vi "WPI_CameraIPCameraRead - Copy.vi"(0 "Refnum in":T1, 1 "Operation":enum16{"Read", "Reopen", "Close"}(ring), 2 "port":u16=80, 5 "address":string, 7 "cgi string":string, 11 "error in (no error)":errorcluster, 13 "Authenticate":bool=TRUE) -> (4 "Refnum out":T1, 6 "length":i32, 10 "Reconnect":bool, 15 "error out":errorcluster)   [LabVIEW 2018]
uses:
  <vilib>/vision/Image Controls.llb/IMAQ Image.ctl
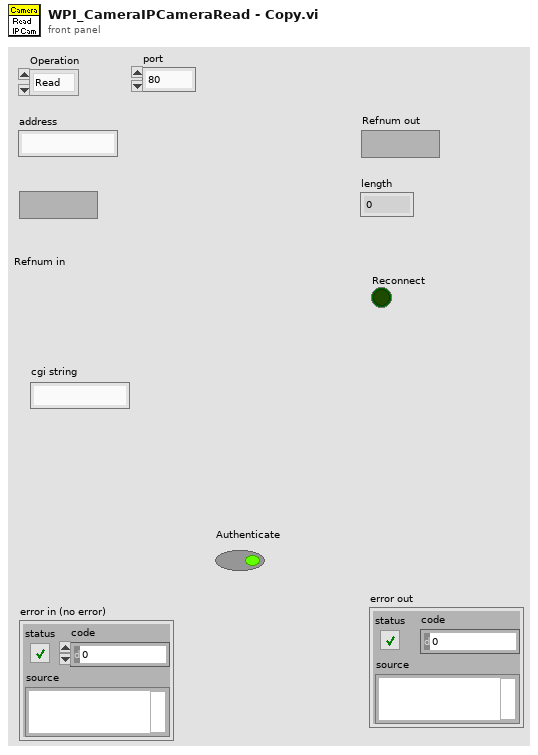
[diagram p1: front panel]
types:
  T1 = typedef "IMAQ Image.ctl" = refnum<image>
  T2 = enum16{"Standard", "Buffered", "CRLF", "Immediate"}
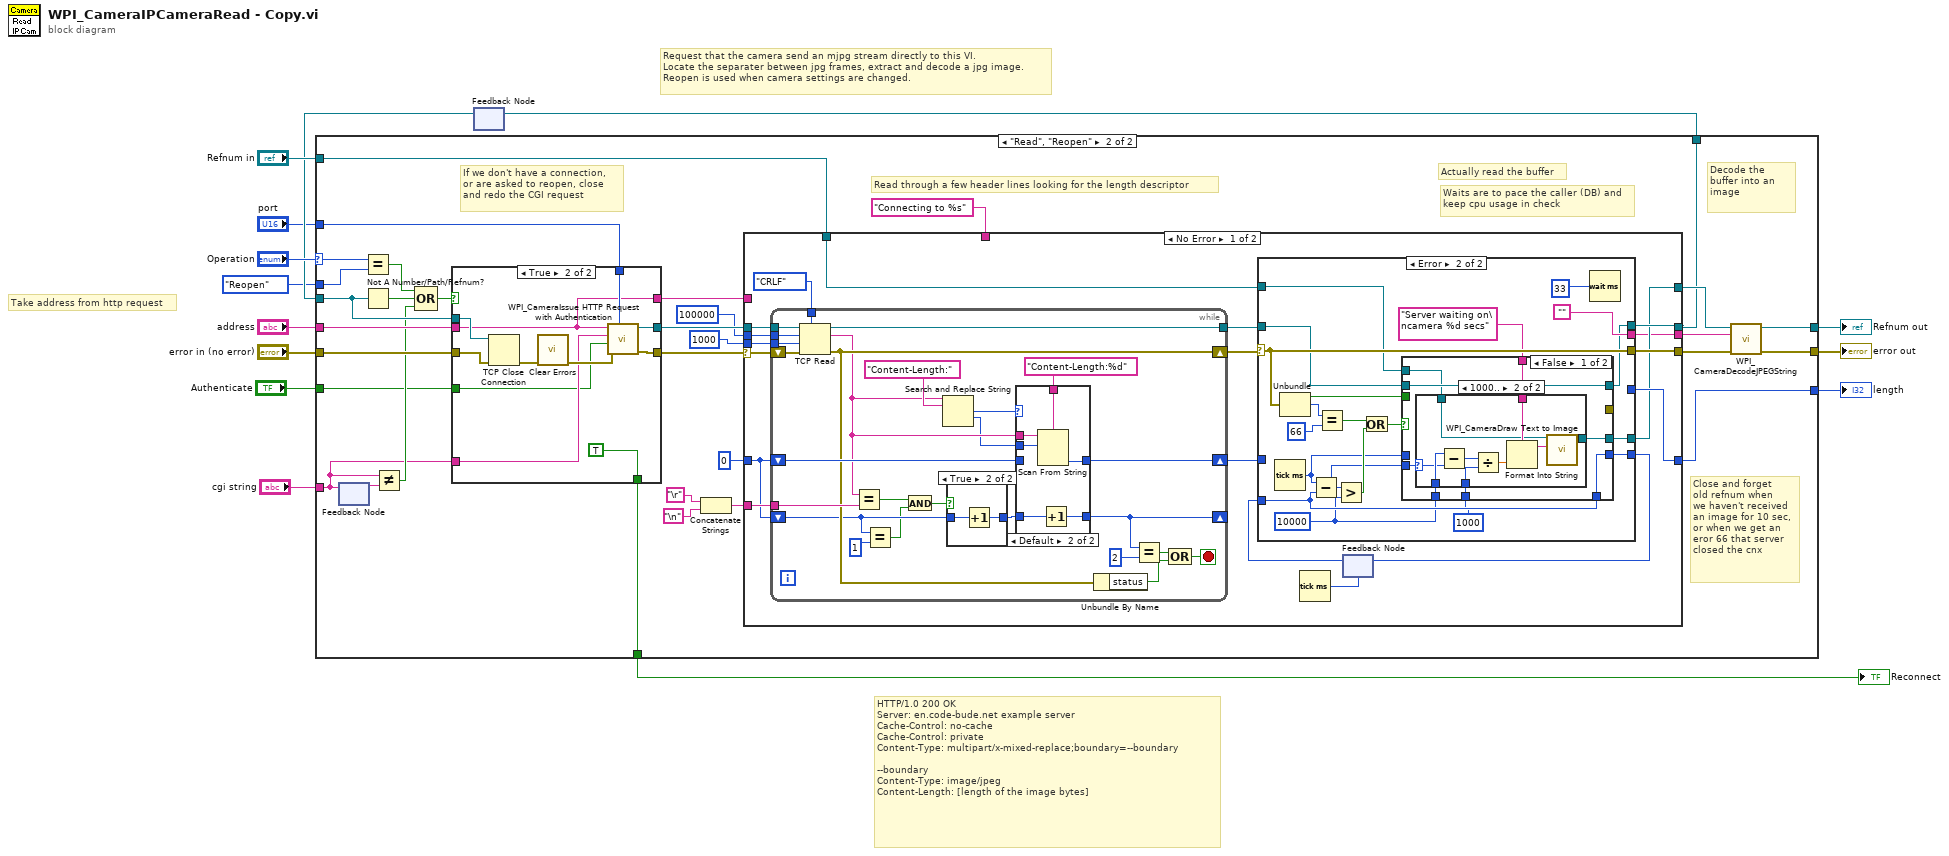
[diagram p0: block diagram]
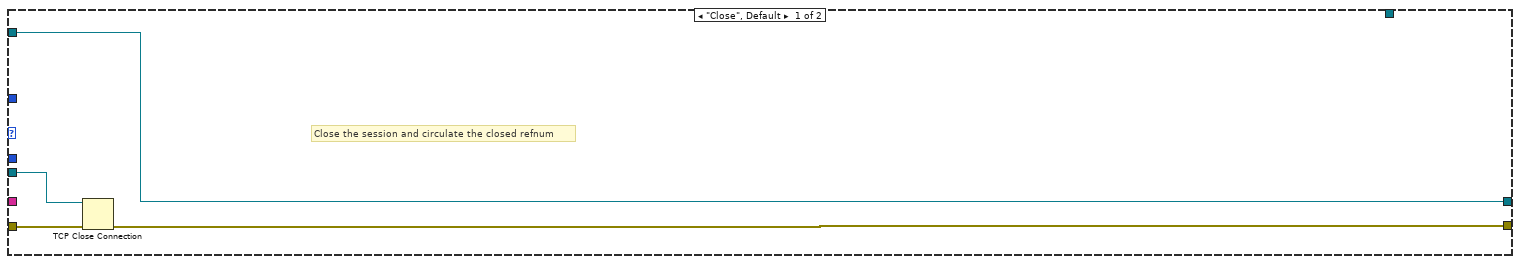
[diagram p2: hidden frame]
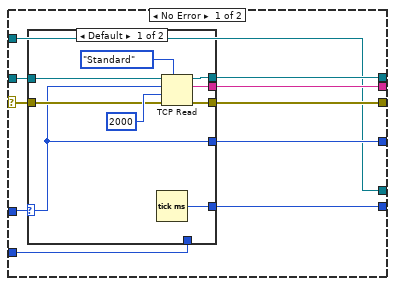
[diagram p4: hidden frame]
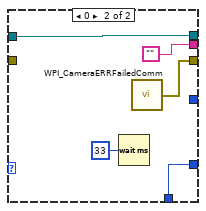
[diagram p5: hidden frame]
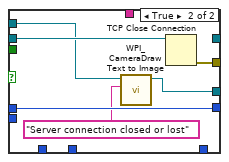
[diagram p7: hidden frame]
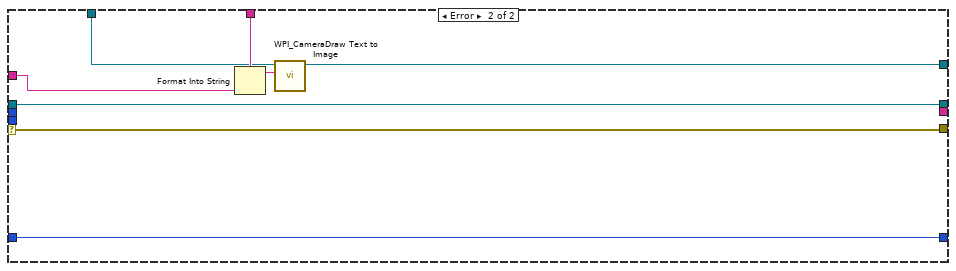
[diagram p10: hidden frame]
diagram:
  # "HTTP/1.0 200 OK\nServer: en.code-bude.net example server\nCache-Control: no-cache\nCache-Control: private\nContent-Type: multipart/x-mixed-replace;boundary=--boundary\n \n--boundary\nContent-Type: image/jpeg\nContent-Length: [length of the image bytes]"
  # "Take address from http request"
  # "Request that the camera send an mjpg stream directly to this VI.\nLocate the separater between jpg frames, extract and decode a jpg image.\nReopen is used when camera settings are changed."
  n1 = feedback #1() -> (w11:refnum<k5>)  [unwired: 1 out]
  n2 = case shown="\"Read\", \"Reopen\"" "Operation" {
    selector: "Operation" -> [_ w38]
    tunnel: "error in (no error)" -> [w17 w44]
    tunnel: "address" -> [_ w43]
    tunnel: [_ w23] -> w8
    tunnel: "cgi string" -> [_ w30]
    tunnel: [w15 w41] -> w9
    tunnel: [w16 w40] -> w10
    tunnel: w11 -> [w18 w39]
    tunnel: "Refnum in" -> [w15 w26]
    tunnel: [_ w22] -> w14
    tunnel: enum16{"Read", "Reopen", "Close"}."Reopen" ("Operation") -> [_ w32]
    tunnel: "port" -> [_ w31]
    tunnel: "Authenticate" -> [_ w28]
    tunnel: [_ w19] -> w1
    frame "Close", Default {
      # "Close the session and circulate the closed refnum"
      n3 = TCP Close Connection(connection ID=w18, error in (no error)=w17) -> (error out=w16:errorcluster)  [unwired: 2 out]
    }
    frame "Read", "Reopen" {
      # "Waits are to pace the caller (DB) and\nkeep cpu usage in check"
      # "Close and forget\nold refnum when\nwe haven't received\nan image for 10 sec,\nor when we get an\neror 66 that server\nclosed the cnx"
      # "Decode the buffer into an image"
      # "Actually read the buffer"
      # "Read through a few header lines looking for the length descriptor"
      # "If we don't have a connection,\nor are asked to reopen, close\nand redo the CGI request"
      n4 = feedback #2() -> (w37:string)  [unwired: 1 out]
      n5 = feedback-in #2(w30) -> ()
      n6 = Equal?(x=w38, y=w32) -> (x = y?=w36:bool)
      n7 = Not A Number/Path/Refnum?(number/path/refnum=w39) -> (NaN/Path/Refnum?=w35:bool)
      n8 = Not Equal?(x=w30, y=w37) -> (x != y?=w33:bool)
      n9 = Compound Arithmetic op=OR(w36, w35, w33) -> (w34:bool)
      n10 = case shown="True" w34 {
        tunnel: [w52 w63] -> w47
        tunnel: [w53 w64] -> w46
        tunnel: w44 -> [w52 w61]
        tunnel: w43 -> [w51 w55]
        tunnel: w39 -> [w53 w62]
        tunnel: w31 -> [_ w58]
        tunnel: w30 -> [_ w57]
        tunnel: w28 -> [_ w56]
        tunnel: [w51 w55] -> w25
        tunnel: [_ TRUE] -> w19
        frame False {
        }
        frame True {
          n11 = TCP Close Connection(connection ID=w62, error in (no error)=w61) -> (error out=w60:errorcluster)  [unwired: 2 out]
          n12 = call <vilib>:"Clear Errors.vi"("error in (no error)"=w60) -> ("error out"=w59:errorcluster)  [unwired: 1 in, 5 out]
          n13 = call <vilib>:"WPI_CameraIssue HTTP Request with Authentication.vi"("port"=w58, "error in (no error)"=w59, "Authenticate"=w56, "Request"=w57, "address"=w55) -> ("error out"=w63:errorcluster, "connection ID (dup)"=w64:refnum<k5>)  [unwired: 5 out]
        }
      }
      n14 = Concatenate Strings("\r", "\n") -> (w48:string)
      n15 = case shown="No Error" w47 {
        selector: w47 -> [w79 w195]
        tunnel: [w68 w195] -> w21
        tunnel: [w69 w194] -> w22
        tunnel: [w67 w196] -> w23
        tunnel: w48 -> [w83 _]
        tunnel: w46 -> [w81 w196]
        tunnel: 1000 ("bytes to read") -> [w80 _]
        tunnel: 0 -> [w78 w194]
        tunnel: 100000 ("bytes to read") -> [w77 _]
        tunnel: [w66 w192] -> w24
        tunnel: "Connecting to %s" ("regular expression") -> [_ w191]
        tunnel: w26 -> [w73 w190]
        tunnel: w25 -> [_ w189]
        tunnel: [w65 _] -> w20
        frame No Error {
          n16 = while {
            tunnel: w81 -> [w177]
            tunnel: [w176] -> w72
            shift-right: [w175] -> w70
            shift-left: w78 -> [w174]
            shift-right: [w157] -> _
            shift-left: w78 -> [w155]
            tunnel: w83 -> [w172]
            tunnel: w80 -> [w162]
            tunnel: T2."CRLF" ("mode (standard)") -> [w171]
            shift-right: [w169] -> w71
            shift-left: w79 -> [w170]
            tunnel: w77 -> [w160]
            stop <- w168 stop-if-true
            n17 = TCP Read(connection ID=w177, bytes to read=w160, error in (no error)=w170, 7:w171, 9:w162) -> (connection ID out=w176:refnum<k5>, data out=w163:string, error out=w169:errorcluster)
            n18 = Equal?(x=w163, y=w172) -> (x = y?=w153:bool)
            n19 = Equal?(x=w155, y=1) -> (x = y?=w154:bool)
            n20 = And(x=w153, y=w154) -> (x .and. y?=w152:bool)
            n21 = Search and Replace String(input string=w163, search string="Content-Length:" ("regular expression")) -> (number of replacements=w167:i32, offset past replacement=w161:i32)  [unwired: 1 in, 7 out]
            n22 = case shown="True" w152 {
              tunnel: w155 -> [w178 w180]
              tunnel: [w178 w179] -> w158
              frame False {
              }
              frame True {
                n23 = Increment(x=w180) -> (x+1=w179:i32)
              }
            }
            n24 = case shown="Default" w167 {
              tunnel: [w182 w188] -> w175
              tunnel: w174 -> [w182 _]
              tunnel: w163 -> [_ w187]
              tunnel: w161 -> [_ w186]
              tunnel: "Content-Length:%d" ("regular expression") -> [_ w185]
              tunnel: w158 -> [w181 w184]
              tunnel: [w181 w183] -> w157
              frame 0 {
              }
              frame Default {
                n25 = Scan From String(format string=w185, input string=w187, initial scan location=w186) -> (output 1=w188:i32)  [unwired: 1 in, 4 out]
                n26 = Increment(x=w184) -> (x+1=w183:i32)
              }
            }
            n27 = Unbundle By Name(w169) -> ("status"=w164:bool)
            n28 = Equal?(x=w157, y=2) -> (x = y?=w165:bool)
            n29 = Compound Arithmetic op=OR(w165, w164) -> (w168:bool)
          }
          n30 = Tick Count (ms)() -> (millisecond timer value=w74:u32)
          n31 = feedback #3(w74) -> (w75:u32)
          n32 = case shown="Error" w71 {
            selector: w71 -> [w89 w126]
            tunnel: [w93 w126] -> w68
            tunnel: [w92 ""] -> w65
            tunnel: [w91 w123] -> w67
            tunnel: w70 -> [w88 _]
            tunnel: w72 -> [w90 w124]
            tunnel: [w87 w117] -> w76
            tunnel: w75 -> [w86 w115]
            tunnel: [w85 _] -> w69
            tunnel: [w84 w109] -> w66
            tunnel: w73 -> [w84 w108]
            frame No Error {
              n33 = case shown="Default" w88 {
                selector: w88 -> [w94 _]
                tunnel: w90 -> [w102 w106]
                tunnel: [w101 w105] -> w93
                tunnel: [w98 ""] -> w92
                tunnel: [w97 w106] -> w91
                tunnel: w89 -> [w96 _]
                tunnel: [w95 w103] -> w87
                tunnel: w86 -> [_ w103]
                tunnel: [w94 _] -> w85
                frame Default {
                  n34 = Tick Count (ms)() -> (millisecond timer value=w95:u32)
                  n35 = TCP Read(connection ID=w102, bytes to read=w94, error in (no error)=w96, 7:T2."Standard" ("mode (standard)"), 9:2000 ("timeout ms (25000)")) -> (connection ID out=w97:refnum<k5>, data out=w98:string, error out=w101:errorcluster)
                }
                frame 0 {
                  n36 = Wait (ms)(milliseconds to wait=u32 33) -> ()  [unwired: 1 out]
                  n37 = call <vilib>:"WPI_CameraERRFailedComm.vi"() -> ("error out"=w105:errorcluster)
                }
              }
            }
            frame Error {
              w112 = u32 10000 ("milliseconds to wait")
              n38 = Tick Count (ms)() -> (millisecond timer value=w116:u32)
              n39 = Unbundle(w126) -> ("status"=w125:bool, "code"=w121:i32)  [unwired: 1 out]
              n40 = Subtract(x=w116, y=w115) -> (x-y=w113:u32)
              n41 = Equal?(x=w121, y=u32 66 ("milliseconds to wait")) -> (x = y?=w120:bool)
              n42 = Greater?(x=w113, y=w112) -> (0:w118:bool)
              n43 = Or(x=w120, y=w118) -> (x .or. y?=w119:bool)
              n44 = case shown="False" w119 {
                tunnel: w125 -> [_ _]
                tunnel: w124 -> [w135 w151]
                tunnel: [w135 _] -> w123
                tunnel: [w134 w150] -> w117
                tunnel: w116 -> [_ w150]
                tunnel: w115 -> [w134 _]
                tunnel: [_ w149] -> _
                tunnel: w113 -> [w133 _]
                tunnel: w112 -> [w132 _]
                tunnel: u32 1000 ("milliseconds to wait") -> [w131 _]
                tunnel: "Server waiting on\ncamera %d secs" ("regular expression") -> [w130 _]
                tunnel: [w129 w148] -> w109
                tunnel: w108 -> [w128 w147]
                frame False {
                  n45 = case shown="1000.." w133 {
                    selector: w133 -> [_ w144]
                    tunnel: w132 -> [_ w145]
                    tunnel: w131 -> [_ w142]
                    tunnel: w130 -> [_ w140]
                    tunnel: [w136 w138] -> w129
                    tunnel: w128 -> [w136 w137]
                    frame 0, Default {
                    }
                    frame 1000.. {
                      n46 = Subtract(x=w145, y=w144) -> (x-y=w143:u32)
                      n47 = Divide(x=w143, y=w142) -> (x/y=w141:dbl)
                      n48 = Format Into String(format string=w140, w141) -> (resulting string=w139:string)  [unwired: 2 in, 1 out]
                      n49 = call <vilib>:"WPI_CameraDraw Text to Image.vi"("Text"=w139, "Refnum in"=w137) -> ("Refnum out"=w138:T1)  [unwired: 9 in]
                    }
                  }
                }
                frame True {
                  n50 = call <vilib>:"WPI_CameraDraw Text to Image.vi"("Text"="Server connection closed or lost" ("regular expression"), "Refnum in"=w147) -> ("Refnum out"=w148:T1)  [unwired: 9 in]
                  n51 = TCP Close Connection(connection ID=w151) -> (error out=w149:errorcluster)  [unwired: 1 in, 2 out]
                }
              }
              n52 = Wait (ms)(milliseconds to wait=u32 33) -> ()  [unwired: 1 out]
            }
          }
          n53 = feedback-in #3(w76) -> ()
        }
        frame Error {
          n54 = Format Into String(format string=w191, w189) -> (resulting string=w193:string)  [unwired: 2 in, 1 out]
          n55 = call <vilib>:"WPI_CameraDraw Text to Image.vi"("Text"=w193, "Refnum in"=w190) -> ("Refnum out"=w192:T1)  [unwired: 9 in]
        }
      }
      n56 = call <vilib>:"WPI_CameraDecodeJPEGString.vi"("error in"=w21, "Compressed Image"=w20, "Image In"=w24) -> ("error out"=w40:errorcluster, "Image Out"=w41:T1)  [unwired: 3 out]
    }
  }
  "length" <- w14
  "error out" <- w10
  "Refnum out" <- w9
  "Reconnect" <- w1
  n57 = feedback-in #1(w8) -> ()
